vi "Do.vi"(8 "error in (no error)":errorcluster, 10 "FormulaG API":refnum<class "FormulaG API.lvclass">, 11 "Pause Cmd in":refnum<class "Pause Cmd.lvclass">) -> (0 "error out":errorcluster, 3 "Pause Cmd out":refnum<class "Pause Cmd.lvclass">)   [LabVIEW 2024, in "FormulaG.lvlib" / "Pause Cmd.lvclass"]
uses:
  Pause Cmd.lvclass
  FormulaG API/FormulaG API.lvclass
  Pause Cmd.lvclass/Pause Cmd.ctl
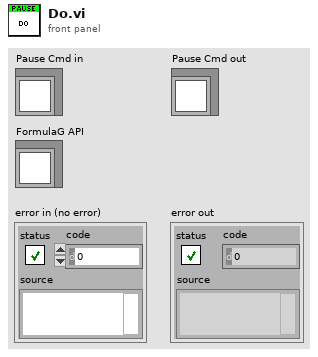
[diagram p1: front panel]
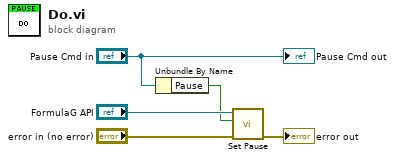
[diagram p0: block diagram]
diagram:
  n1 = Unbundle By Name("Pause Cmd in") -> ("Pause"=w3:bool)
  n2 = call "Set Pause.vi"("error in (no error)"="error in (no error)", "Pause"=w3, "FormulaG API in"="FormulaG API") -> ("error out"=→"error out":errorcluster)  [unwired: 7 in, 1 out]
  "Pause Cmd out" <- "Pause Cmd in"
